vi "hPID.vi"(6 "ID":string, 7 "LabVIEW Web Service Request":refnum<class "Web Request.lvclass">, 9 "D":dbl, 10 "I":dbl, 11 "P":dbl) -> ()   [LabVIEW 2014]
uses:
  <vilib>/wsapi/Web Request.lvclass
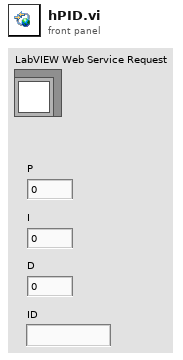
[diagram p1: front panel]
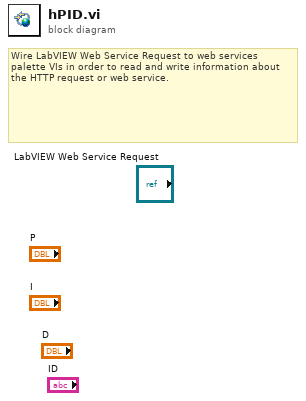
[diagram p0: block diagram]
diagram:
  # "Wire LabVIEW Web Service Request to web services palette VIs in order to read and write information about the HTTP request or web service."
